vi "GObject to .NET Object.vi"(8 "error in (no error)":errorcluster, 10 "G Object":variant) -> (0 "error out":errorcluster, 2 ".NET Object":refnum<k24>)   [LabVIEW 2018, in "G .NET.lvlib"]
uses:
  G .NET.lvlib
  <vilib>/Utility/Data Type/NI_Data Type.lvlib
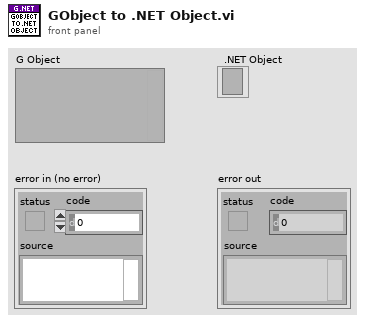
[diagram p1: front panel]
types:
  T1 = typedef "NI_Data Type.lvlib/Data Type.ctl" = enum8{"Invalid Type", "Void", "I8", "I16", "I32", "I64", "U8", "U16", "U32", "U64", "Single Float", "Double Float", "Extended Float", "Single Complex", "Double Complex", "Extended Complex", "Enum U8", "Enum U16", "Enum U32", "Enum U64", "Single Float With Unit", "Double Float With Unit", "Extended Float With Unit", "Single Complex with Unit", "Double Complex with Unit", "Extended Complex with Unit", "Boolean", "String", "Path", "Picture", "Tag", "Array", "Cluster", "Variant", "LV Variant", "Waveform", "Timestamp", "Digital Waveform", "Digital Data", "ExpressData", "Refnum", "External Data", "VI", "Poly VI", "LabVIEW Class Instance", "Fixed Point"}
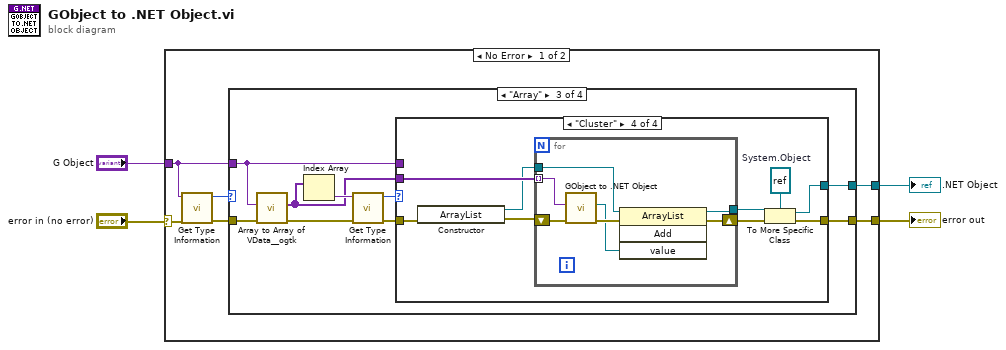
[diagram p0: block diagram]
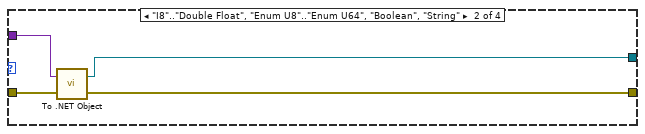
[diagram p3: hidden frame]
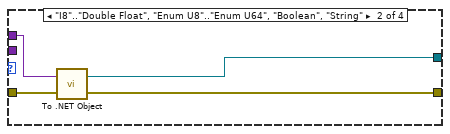
[diagram p5: hidden frame]
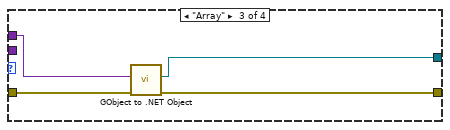
[diagram p6: hidden frame]
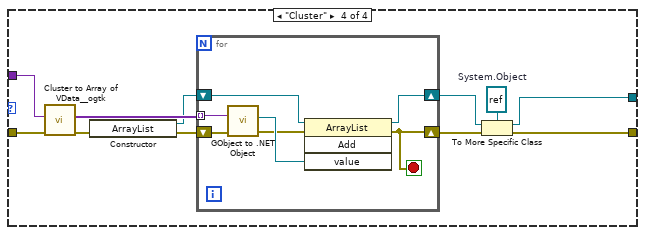
[diagram p7: hidden frame]
diagram:
  n1 = case shown="No Error" "error in (no error)" {
    selector: "error in (no error)" -> [w6 w68]
    tunnel: "G Object" -> [w9 _]
    tunnel: [w8 w68] -> w3
    tunnel: [w7 _] -> w2
    frame No Error {
      n2 = call <vilib>:"Get Type Information.vi"("error in (no error)"=w6, "Variant"=w9) -> ("error out"=w10:errorcluster, "Type"=w5:T1)  [unwired: 5 in, 3 out]
      n3 = case shown="\"Array\"" w5 {
        tunnel: w10 -> [w11 w15 w24 w60]
        tunnel: w9 -> [_ w14 w19 w59]
        tunnel: [w11 w13 w18 w52] -> w8
        tunnel: [_ w12 w17 w50] -> w7
        frame Default {
        }
        frame "I8".."Double Float", "Enum U8".."Enum U64", "Boolean", "String" {
          n4 = call <vilib>:"To .NET Object.vi"("error in (no error)"=w15, "anything"=w14) -> ("error out"=w13:errorcluster, ".NET object"=w12:refnum<k24>)
        }
        frame "Array" {
          n5 = call <userlib>:"Array to Array of VData__ogtk.vi"("error in (no error)"=w24, "MultiD Array"=w19) -> ("error out"=w22:errorcluster, "1D Array of Variants"=w16:variant[])  [unwired: 8 in]
          n6 = Index Array(array=w16) -> (element=w23:variant)  [unwired: 1 in]
          n7 = call <vilib>:"Get Type Information.vi"("error in (no error)"=w22, "Variant"=w23) -> ("error out"=w21:errorcluster, "Type"=w20:T1)  [unwired: 5 in, 3 out]
          n8 = case shown="\"Cluster\"" w20 {
            tunnel: w21 -> [w25 w29 w33 w36]
            tunnel: w19 -> [_ w28 w32 _]
            tunnel: [w25 w27 w30 w38] -> w18
            tunnel: [_ w26 w31 w39] -> w17
            tunnel: w16 -> [_ _ _ w37]
            frame Default {
            }
            frame "I8".."Double Float", "Enum U8".."Enum U64", "Boolean", "String" {
              n9 = call <vilib>:"To .NET Object.vi"("error in (no error)"=w29, "anything"=w28) -> ("error out"=w27:errorcluster, ".NET object"=w26:refnum<k24>)
            }
            frame "Array" {
              n10 = call "GObject to .NET Object.vi"("error in (no error)"=w33, "G Object"=w32) -> ("error out"=w30:errorcluster, ".NET Object"=w31:refnum<k24>)  [unwired: 8 in]
            }
            frame "Cluster" {
              w40 = refnum<k24> refnum  # System.Object
              n11 = constructor class="ArrayList"(error in=w36) -> (reference out=w34:refnum<k24>, error out=w35:errorcluster)  [unwired: 2 in, 1 out]
              n12 = for {
                tunnel: w37 -> [w49] mode=indexing
                shift-right: [w47] -> w42
                shift-left: w35 -> [w48]
                tunnel: [w45] -> w41
                tunnel: w34 -> [w44]
                n13 = call "GObject to .NET Object.vi"("error in (no error)"=w48, "G Object"=w49) -> ("error out"=w46:errorcluster, ".NET Object"=w43:refnum<k24>)  [unwired: 8 in]
                n14 = invoke class="ArrayList" method="Add"(reference=w44, error in=w46, "value"=w43) -> (reference out=w45:refnum<k24>, error out=w47:errorcluster)  [unwired: 1 in, 2 out]
              }
              n15 = To More Specific Class(target class=w40, reference=w41, error in=w42) -> (specific class reference=w39:refnum<k24>, error out=w38:errorcluster)
            }
          }
        }
        frame "Cluster" {
          w54 = refnum<k24> refnum  # System.Object
          n16 = call <userlib>:"Cluster to Array of VData__ogtk.vi"("error in (no error)"=w60, "Cluster"=w59) -> ("error out"=w58:errorcluster, "Array of VData"=w56:variant[])  [unwired: 8 in]
          n17 = constructor class="ArrayList"(error in=w58) -> (reference out=w55:refnum<k24>, error out=w57:errorcluster)  [unwired: 2 in, 1 out]
          n18 = for {
            shift-right: [w65] -> w53
            shift-left: w57 -> [w64]
            tunnel: w56 -> [w63] mode=indexing
            shift-right: [w66] -> w51
            shift-left: w55 -> [w67]
            stop <- w65 stop-if-true
            n19 = call "GObject to .NET Object.vi"("error in (no error)"=w64, "G Object"=w63) -> ("error out"=w61:errorcluster, ".NET Object"=w62:refnum<k24>)  [unwired: 8 in]
            n20 = invoke class="ArrayList" method="Add"(reference=w67, error in=w61, "value"=w62) -> (reference out=w66:refnum<k24>, error out=w65:errorcluster)  [unwired: 1 in, 2 out]
          }
          n21 = To More Specific Class(target class=w54, reference=w51, error in=w53) -> (specific class reference=w50:refnum<k24>, error out=w52:errorcluster)
        }
      }
    }
    frame Error {
    }
  }
  "error out" <- w3
  ".NET Object" <- w2
